vi "NML Data Acquisition-New.vi"() -> ()   [LabVIEW 2019]
doc: "This VI is designed to scan data each time the the trigger channel changes by an amount ∆ trigger.\nCopyright 2013\nScott Hannahs, NHMFL - FSU, July 2013"
uses:
  Sub Controls/Data Graph.ctl
  Sub Controls/Pause Switch.ctl
  Sub Controls/SystemCheckBox-resize.ctl
  Sub Controls/DataAcq User Events.ctl
panel:
  in  "Show Times":bool
  out "Time (mS)":dbl[](array[numeric])
  out "Logo":u16(ring)=2
  in  "ColorSelector":bool[](array[boolean])
  out "File Ref Num":refnum<file>
  out "All Data":dbl[][](array[numeric])
  out "Data":dbl[](array[numeric])=[nan, nan] format="%_4e"
  in  "Labels":string[](array[string])=["Field", "Timestamp"]
  out "Colors":u32[](array[colorbox])=[16748168, 2796287]
  out "# Data Points":i32
  in  "Comments":string="This data's for you!\n"
  in  "User Name":string="Conan The Scientist"
  in  "File Name":string="Test"
  in  "Open BD":bool
  in  "Pause":T1=TRUE
  in  "∆ Trigger":dbl min=0.0 format="%.3f"
  in  "Trigger Column":u32(ring) items=["Time", "Field", "Timestamp"]
  in  "Print":bool
  in  "Quit":bool
  in  "New/Stop":bool
  in  "Test":bool
  in  "Show Help":bool
  in  "Configure":bool
  in  "X-Axis":u32(ring)=1 items=["Point #", "Field", "Timestamp"]
  out "Data Plot":T2
  in  "Offset":dbl[](array[numeric])=[0.0, 0.0] format="%^_3e"
  in  "Display":T3[](array[typedef])=[TRUE, TRUE]
  in  "Scale":dbl[](array[numeric])=[1.0, 1.0] format="%^_3e"
  out "Status":string="Standby"
  # "NHMFL Data Acqusition System V 2.4.1\nScott Hannahs"
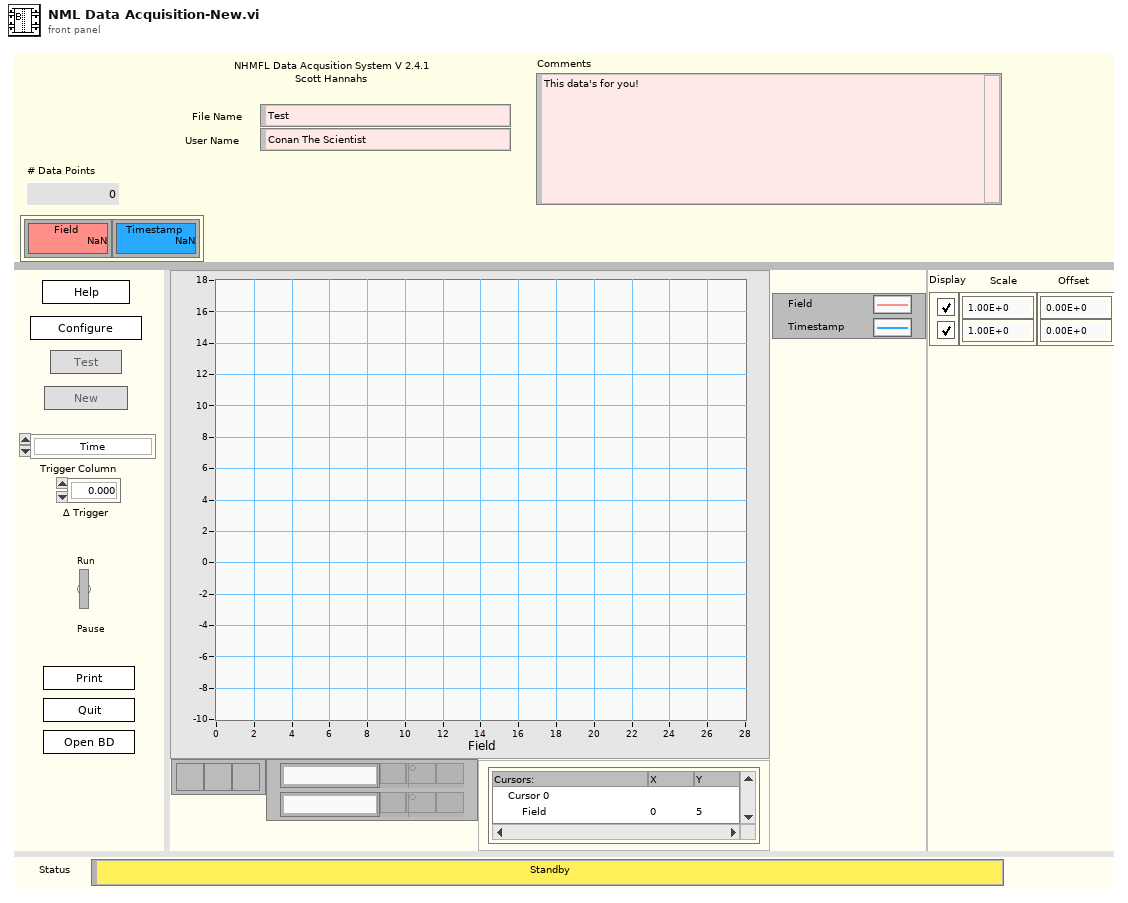
[diagram p1: front panel]
types:
  T1 = typedef "Pause Switch.ctl" = bool
  T2 = typedef "Data Graph.ctl" = cluster{dbl[], dbl[]}[]
  T3 = typedef "SystemCheckBox-resize.ctl" = bool
  T4 = typedef "DataAcq User Events.ctl" = enum16{"Update Data Display", "Store Data"}
  T5 = enum8{"Enabled", "Disabled", "Disabled and Grayed Out"}
  T6 = typedef "Instrument Properties.ctl" = cluster{"Public":T7, "Private":T8}
  T7 = typedef "Public.ctl" = cluster{"Column Name":string[], "Trace Color":u32[]}
  T8 = typedef "Private.ctl" = cluster{"Path":path, "VI Refnum":T9, "Name":string, "# of Values":i32, "Scale Factors":dbl[], "Display":T3[], "Offset":dbl[]}
  T9 = typedef "Instrument Ref.ctl" = refnum<vi>
  T10 = typedef "LVRectTypeDef.ctl" = cluster{"Left":i16, "Top":i16, "Right":i16, "Bottom":i16}
  T11 = typedef "LVPositionTypeDef.ctl" = cluster{"Left":i32, "Top":i32}
  T12 = typedef "imagedata.ctl" = cluster{"image type":i32, "image depth":i32, "image":u8[], "mask":u8[], "colors":u32[], "Rectangle":cluster{"left":i16, "top":i16, "right":i16, "bottom":i16}}
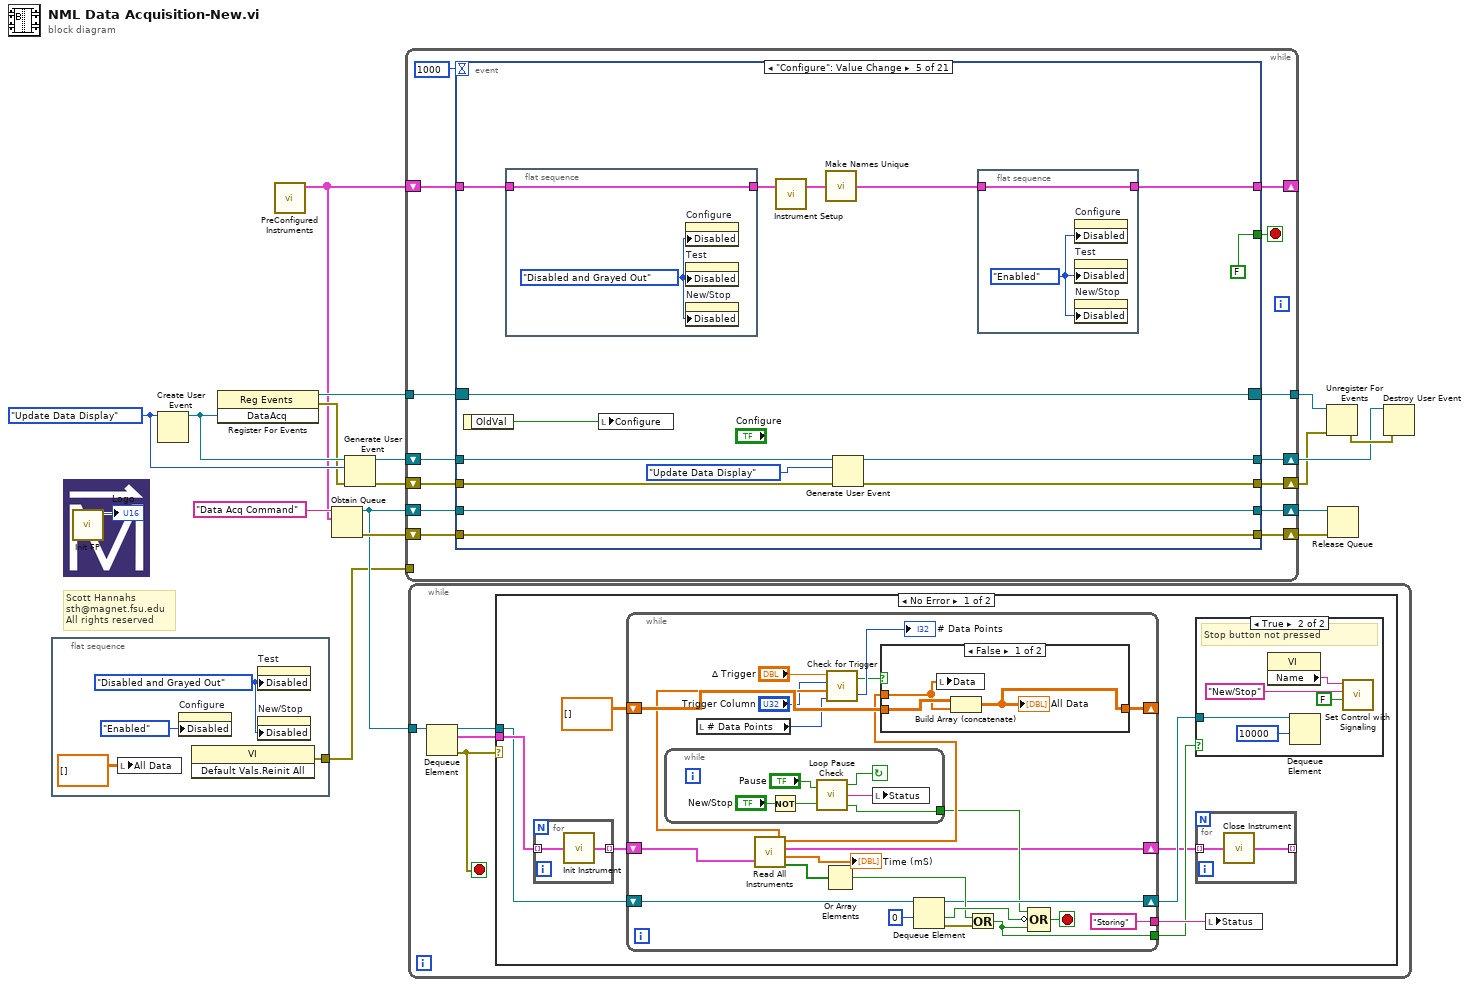
[diagram p0: block diagram]
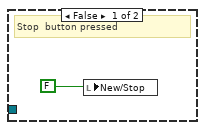
[diagram p2: hidden frame]
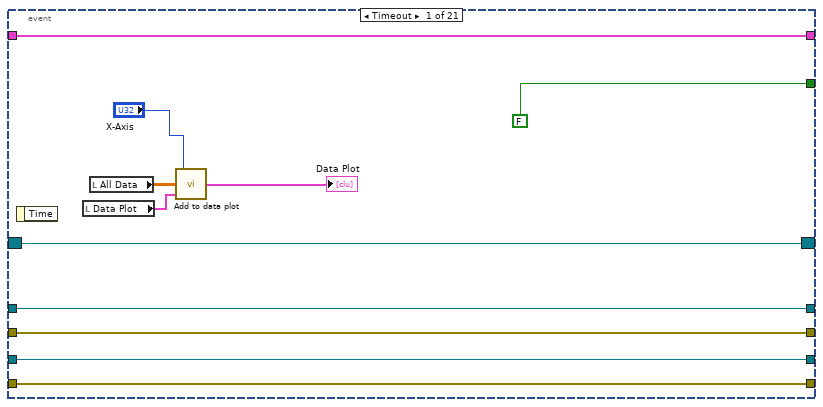
[diagram p5: hidden frame]
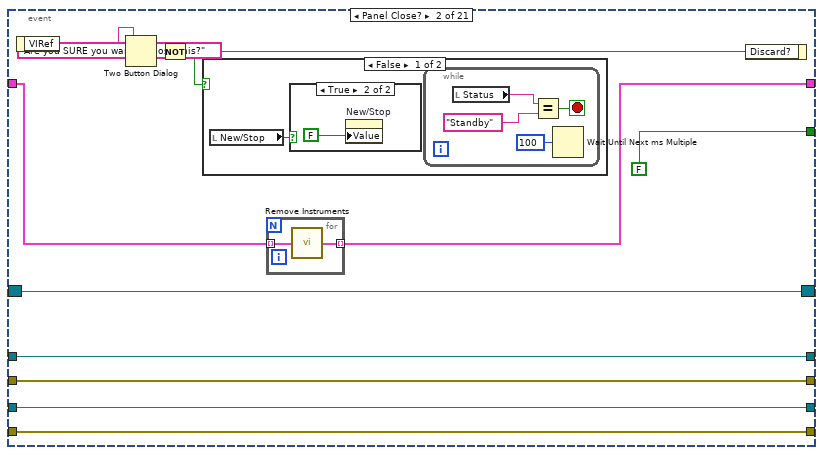
[diagram p6: hidden frame]
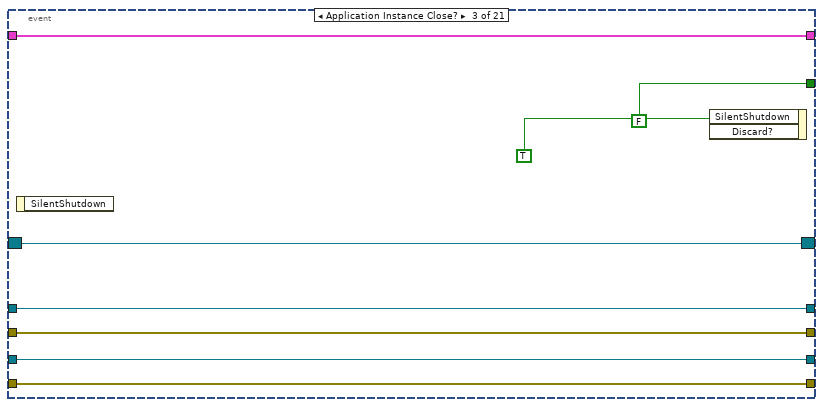
[diagram p9: hidden frame]
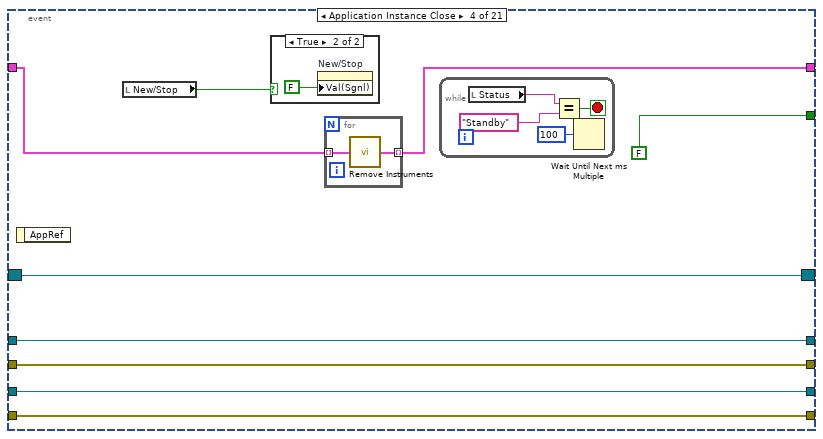
[diagram p10: hidden frame]
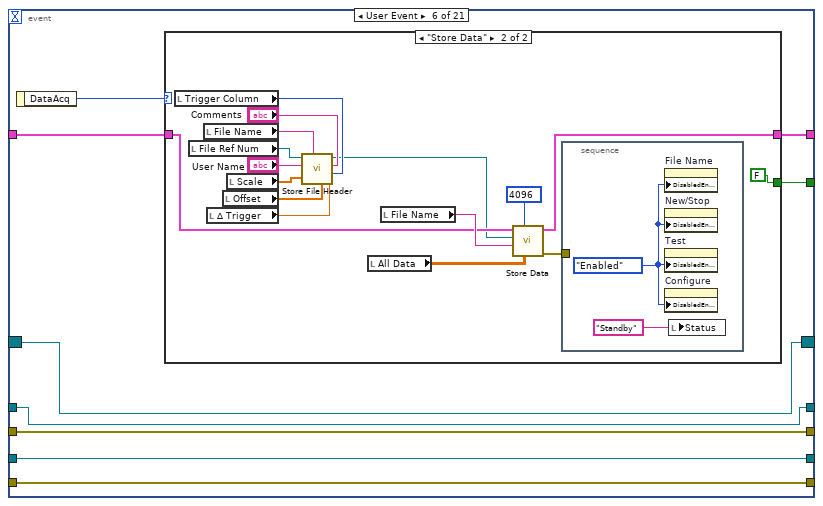
[diagram p12: hidden frame]
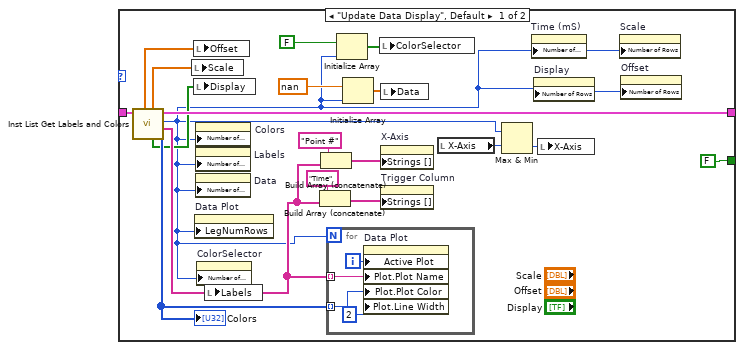
[diagram p13: hidden frame]
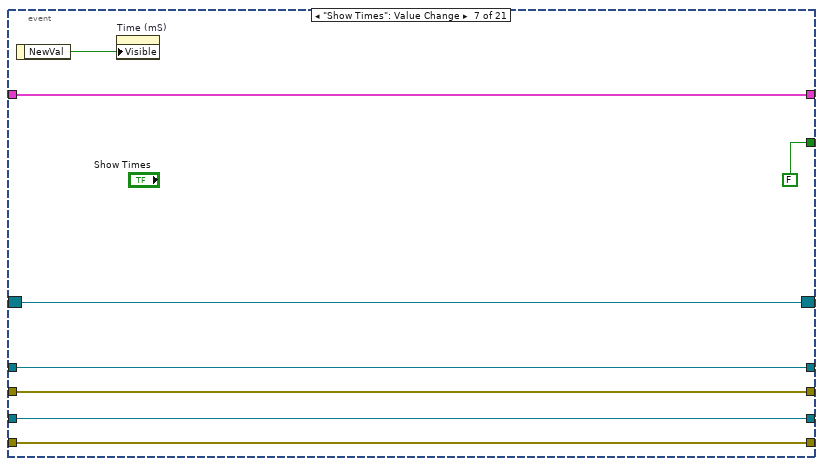
[diagram p14: hidden frame]
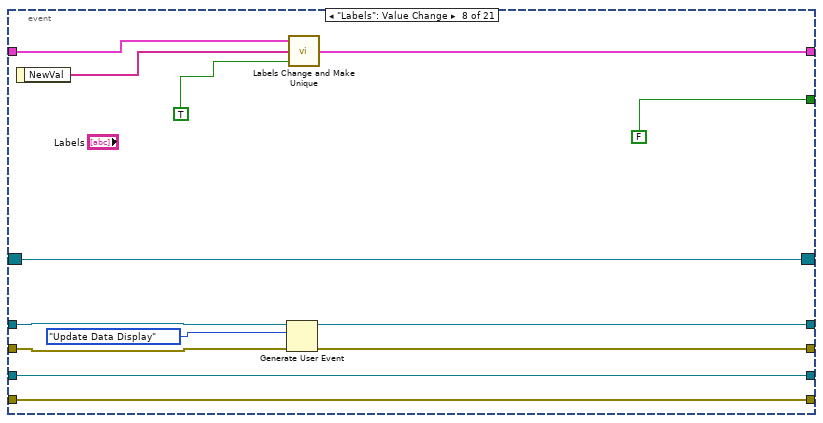
[diagram p15: hidden frame]
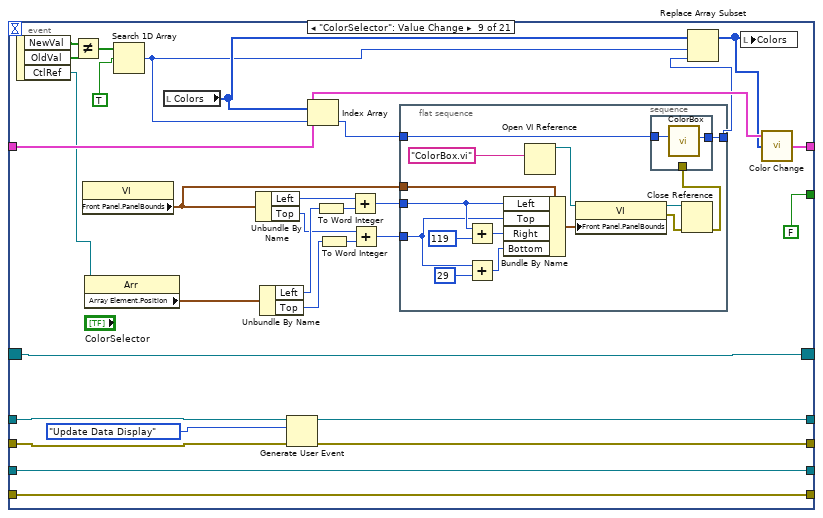
[diagram p16: hidden frame]
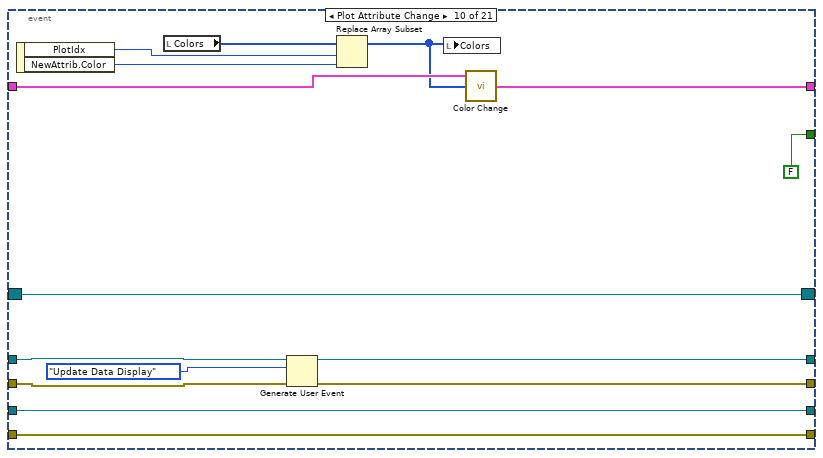
[diagram p17: hidden frame]
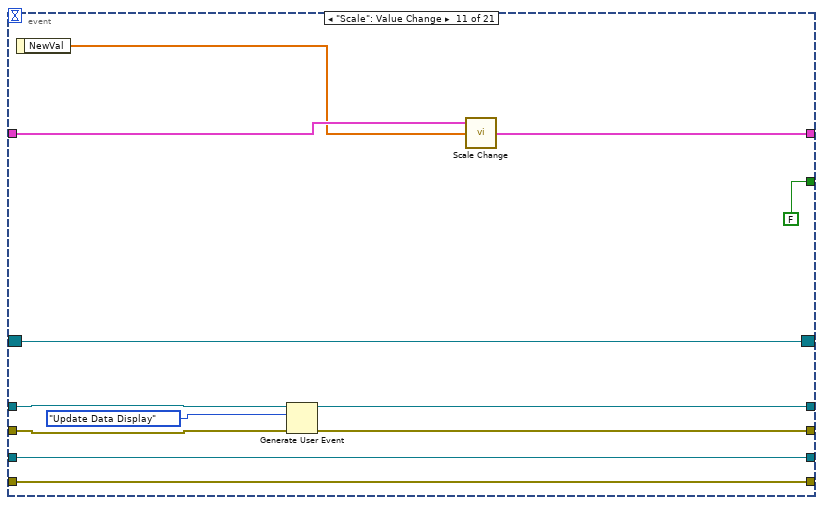
[diagram p18: hidden frame]
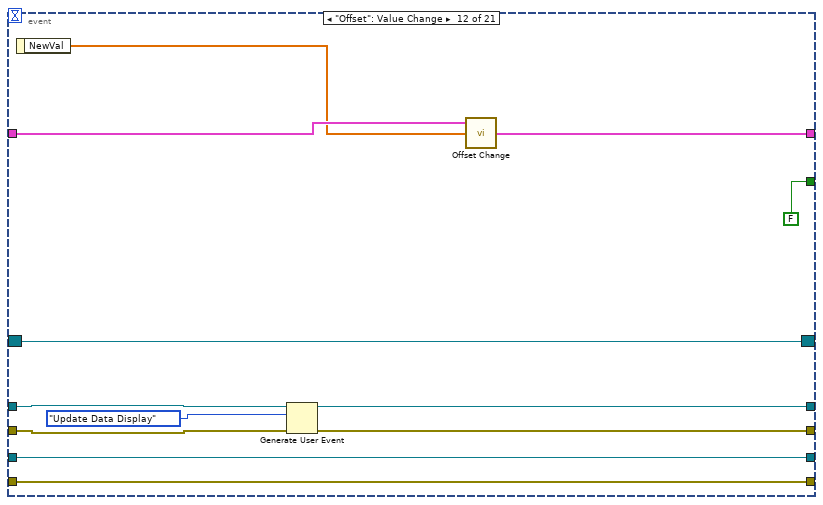
[diagram p19: hidden frame]
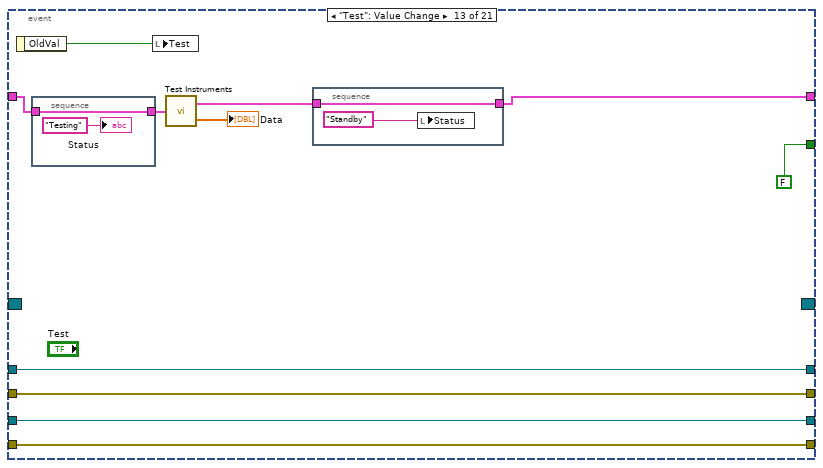
[diagram p20: hidden frame]
diagram:
  w16 = DataAcq_User_Events."Update Data Display" ("DataAcq")
  # "Scott Hannahs\nsth@magnet.fsu.edu\nAll rights reserved"
  n1 = flat-sequence {
    tunnel: [w21] -> w3
    frame #0 {
      w22 = T5."Disabled and Grayed Out" ("Disabled")
      n2 = local write "All Data"(dbl[][] [] ("All Data")) -> ()
      n3 = property on="Configure" class="Bool (strict)"("Disabled"=T5."Enabled") -> ()  [unwired: 2 in, 2 out]
      n4 = invoke class="VI" method="Default Vals.Reinit All"() -> (error out=w21:errorcluster)  [unwired: 3 in, 2 out]
      n5 = property on="Test" class="Bool (strict)"("Disabled"=w22) -> ()  [unwired: 2 in, 2 out]
      n6 = property on="New/Stop" class="Bool (strict)"("Disabled"=w22) -> ()  [unwired: 2 in, 2 out]
    }
  }
  n7 = call "Init FP.vi"() -> ("Logo"=→"Logo":u16)  [unwired: 11 in]
  n8 = Create User Event(user event datatype=w16) -> (user event=w17:refnum<user-event>)  [unwired: 1 in, 1 out]
  n9 = register-events(w17) -> (reference out=w18:refnum<event-registration>, error out=w15:errorcluster)  [unwired: 2 in]
  n10 = call "PreConfigured Instruments.vi"() -> ("PreConfigured Instruments"=w1:T6[])  [unwired: 11 in]
  n11 = Obtain Queue(name (unnamed)="Data Acq Command", element data type=w1) -> (queue out=w5:refnum<queue>, error out=w7:errorcluster)  [unwired: 3 in, 1 out]
  n12 = Generate User Event(user event=w17, event data cluster=w16, error in=w15) -> (user event out=w14:refnum<user-event>, error out=w9:errorcluster)  [unwired: 1 in]
  n13 = while {
    shift-right: [w35] -> _
    shift-left: w1 -> [w34]
    tunnel: w18 -> [w33]
    shift-right: [w31] -> w11
    shift-left: w14 -> [w32]
    tunnel: [w30] -> w13
    shift-right: [w28] -> w10
    shift-left: w5 -> [w29]
    shift-right: [w26] -> w8
    shift-left: w9 -> [w27]
    shift-right: [w24] -> w6
    shift-left: w7 -> [w25]
    tunnel: w3 -> [_]
    stop <- w36 stop-if-true
    n14 = event shown="[4] \"Configure\": Value Change" {
      selector: w33 -> [w38 w48 w67 w75 w96 w110 w164 w176 w209 w241 w253 w265 _ w288 w356 w365 w383 w398 w435 w444 w461]
      dyn-events: [w38 w48 w67 w75 w96 w110 w164 w176 w209 w241 w253 w265 _ w288 w356 w365 w383 w398 w435 w444 w461] -> w30
      timeout: 1000 -> [_ _ _ _ _ _ _ _ _ _ _ _ _ _ _ _ _ _ _ _ _]
      tunnel: [FALSE ("NewVal") FALSE ("NewVal") FALSE ("NewVal") FALSE ("NewVal") FALSE ("stop") w118 FALSE ("NewVal") FALSE ("NewVal") FALSE ("NewVal") FALSE ("NewVal") FALSE ("NewVal") FALSE ("NewVal") FALSE ("stop") FALSE ("stop") FALSE ("stop") FALSE ("stop") FALSE ("stop") FALSE ("NewVal") FALSE ("NewVal") w443 FALSE ("NewVal")] -> w36
      tunnel: w34 -> [w41 w54 w68 w77 w95 w116 w166 w180 w197 w233 w245 w257 w273 w292 w357 w371 w382 w408 w440 w450 w463]
      tunnel: [w41 w53 w68 w76 w92 w117 w166 w178 w211 w243 w255 w267 w270 w291 w357 w371 w381 w408 w440 w449 w463] -> w35
      tunnel: w32 -> [w45 w52 w72 w81 w104 w115 w163 w171 w205 w237 w249 w261 w277 w296 w359 w373 w390 w404 w439 w448 w460]
      tunnel: [w45 w52 w72 w81 w102 w115 w163 w170 w204 w236 w248 w260 w277 w295 w359 w373 w390 w404 w439 w448 w460] -> w31
      tunnel: [w43 w50 w70 w79 w99 w113 w161 w175 w208 w240 w252 w264 w276 w293 w362 w375 w388 w406 w437 w446 w458] -> w28
      tunnel: w29 -> [w43 w50 w70 w79 w99 w113 w161 w175 w208 w240 w252 w264 w276 w294 w362 w375 w388 w406 w437 w446 w458]
      tunnel: [w44 w51 w71 w80 w101 w114 w162 w169 w203 w235 w247 w259 w275 w286 w360 w376 w389 w405 w438 w447 w459] -> w26
      tunnel: w27 -> [w44 w51 w71 w80 w100 w114 w162 w168 w202 w234 w246 w258 w275 w287 w360 w376 w389 w405 w438 w447 w459]
      tunnel: [w42 w49 w69 w78 w98 w112 w160 w174 w207 w239 w251 w263 w274 w289 w361 w374 w387 w407 w436 w445 w457] -> w24
      tunnel: w25 -> [w42 w49 w69 w78 w98 w112 w160 w174 w207 w239 w251 w263 w274 w290 w361 w374 w387 w407 w436 w445 w457]
      event Timeout {
        n15 = event-data() -> ()  [unwired: 1 in, 1 out]
        n16 = local read "Data Plot"() -> (w37:T2)
        n17 = local read "All Data"() -> (w47:dbl[][])
        n18 = call "Add to data plot.vi"("Data Plot In"=w37, "All Data"=w47, "X-Axis"="X-Axis") -> ("Data PlotOut"=→"Data Plot":T2)
      }
      event Panel Close? {
        n19 = event-data() -> ()  [unwired: 1 in, 1 out]
        n20 = Two Button Dialog(message="Are you SURE you want to close this?") -> (T button?=w58:bool)  [unwired: 2 in]
        n21 = Not(x=w58) -> (.not. x?=w56:bool)
        n22 = case shown="False" w56 {
          frame False {
            n23 = local read "New/Stop"() -> (w61:bool)
            n24 = case shown="True" w61 {
              frame False {
              }
              frame True {
                n25 = property on="New/Stop" class="Bool (strict)"("Value"=FALSE ("New/Stop")) -> ()  [unwired: 2 in, 2 out]
              }
            }
            n26 = while {
              stop <- w65 stop-if-true
              n27 = local read "Status"() -> (w66:string)
              n28 = Equal?(x=w66, y="Standby") -> (x = y?=w65:bool)
              n29 = Wait Until Next ms Multiple(millisecond multiple=u32 100) -> ()  [unwired: 1 out]
            }
          }
          frame True {
          }
        }
        n30 = for {
          tunnel: w54 -> [w60] mode=indexing
          tunnel: [w59] -> w53 mode=indexing
          n31 = call "Remove Instruments.vi"("Instrument Prop"=w60) -> ("Instrument Prop Out"=w59:T6)
        }
        n32 = event-data("Discard?"=w56) -> ()  [unwired: 1 in, 1 out]
      }
      event Application Instance Close? {
        n33 = event-data() -> ()  [unwired: 1 in, 1 out]
        n34 = event-data("SilentShutdown"=TRUE) -> ()  [unwired: 2 in, 1 out]
      }
      event Application Instance Close {
        n35 = event-data() -> ()  [unwired: 1 in, 1 out]
        n36 = local read "New/Stop"() -> (w83:bool)
        n37 = case shown="True" w83 {
          frame False {
          }
          frame True {
            n38 = property on="New/Stop" class="Bool (strict)"("Val(Sgnl)"=FALSE ("New/Stop")) -> ()  [unwired: 2 in, 2 out]
          }
        }
        n39 = for {
          tunnel: w77 -> [w85] mode=indexing
          tunnel: [w84] -> w76 mode=indexing
          n40 = call "Remove Instruments.vi"("Instrument Prop"=w85) -> ("Instrument Prop Out"=w84:T6)
        }
        n41 = while {
          stop <- w89 stop-if-true
          n42 = local read "Status"() -> (w90:string)
          n43 = Equal?(x=w90, y="Standby") -> (x = y?=w89:bool)
          n44 = Wait Until Next ms Multiple(millisecond multiple=u32 100) -> ()  [unwired: 1 out]
        }
      }
      event "Configure": Value Change {
        n45 = event-data() -> ("OldVal"=w91:bool)  [unwired: 1 in]
        n46 = flat-sequence {
          tunnel: [w107] -> w94
          tunnel: w95 -> [w107]
          frame #0 {
            w106 = T5."Disabled and Grayed Out" ("Disabled")
            n47 = property on="Configure" class="Bool (strict)"("Disabled"=w106) -> ()  [unwired: 2 in, 2 out]
            n48 = property on="Test" class="Bool (strict)"("Disabled"=w106) -> ()  [unwired: 2 in, 2 out]
            n49 = property on="New/Stop" class="Bool (strict)"("Disabled"=w106) -> ()  [unwired: 2 in, 2 out]
          }
        }
        n50 = local write "Configure"(w91) -> ()
        n51 = call "Instrument Setup.vi"("Configured Inst"=w94) -> ("Configured Inst dup"=w97:T6[])  [unwired: 2 in]
        n52 = call "Make Names Unique.vi"("Configured Inst"=w97) -> ("Configured Inst dup"=w93:T6[])
        n53 = Generate User Event(user event=w104, event data cluster=DataAcq_User_Events."Update Data Display" ("event data"), error in=w100) -> (user event out=w102:refnum<user-event>, error out=w101:errorcluster)  [unwired: 1 in]
        n54 = flat-sequence {
          tunnel: w93 -> [w109]
          tunnel: [w109] -> w92
          frame #0 {
            w108 = T5."Enabled" ("Disabled")
            n55 = property on="Configure" class="Bool (strict)"("Disabled"=w108) -> ()  [unwired: 2 in, 2 out]
            n56 = property on="Test" class="Bool (strict)"("Disabled"=w108) -> ()  [unwired: 2 in, 2 out]
            n57 = property on="New/Stop" class="Bool (strict)"("Disabled"=w108) -> ()  [unwired: 2 in, 2 out]
          }
        }
      }
      event User Event {
        n58 = event-data() -> ("DataAcq"=w111:T4)  [unwired: 1 in]
        n59 = case shown="\"Store Data\"" w111 {
          tunnel: [FALSE ("stop") FALSE ("stop")] -> w118
          tunnel: [w136 w146] -> w117
          tunnel: w116 -> [w135 w145]
          frame "Update Data Display", Default {
            n60 = call "Inst List Get Labels and Colors.vi"("Instrument List"=w135) -> ("Colors"=w132:u32[], "Labels"=w125:string[], "Number of Columns"=w119:u32, "Instrument List Out"=w136:T6[], "Display"=w121:T3[], "Scale Factors"=w122:dbl[], "Offsets"=w120:dbl[])  [unwired: 4 in]
            "Colors" <- w132
            n61 = local write "Scale"(w122) -> ()
            n62 = local write "Offset"(w120) -> ()
            n63 = local write "Display"(w121) -> ()
            n64 = property on="Data Plot" class="XYGraph (strict)"("LegNumRows"=w119) -> ()  [unwired: 2 in, 2 out]
            n65 = property on="Colors" class="Arr (strict)"("Number of Columns"=w119) -> ()  [unwired: 2 in, 2 out]
            n66 = property on="Labels" class="Arr (strict)"("Number of Columns"=w119) -> ()  [unwired: 2 in, 2 out]
            n67 = property on="Data" class="Arr (strict)"("Number of Columns"=w119) -> ()  [unwired: 2 in, 2 out]
            n68 = property on="ColorSelector" class="Arr"("Number of Columns"=w119) -> ()  [unwired: 2 in, 2 out]
            n69 = local write "Labels"(w125) -> ()
            n70 = Build Array (concatenate)("Time", w125) -> (w131:string[])
            n71 = Build Array (concatenate)("Point #", w125) -> (w129:string[])
            n72 = for {
              N: w119 -> [_]
              tunnel: w125 -> [w139] mode=indexing
              tunnel: w132 -> [w141] mode=indexing
              i -> [w140]
              n73 = property on="Data Plot" class="XYGraph (strict)"("Active Plot"=w140, "Plot.Plot Name"=w139, "Plot.Plot Color"=w141, "Plot.Line Width"=u8 2) -> ()  [unwired: 2 in, 2 out]
            }
            n74 = Initialize Array(FALSE, w119) -> (w123:bool[])
            n75 = Initialize Array(nan, w119) -> (w134:dbl[])
            n76 = local write "ColorSelector"(w123) -> ()
            n77 = local write "Data"(w134) -> ()
            n78 = property on="X-Axis" class="Ring (strict)"("Strings []"=w129) -> ()  [unwired: 2 in, 2 out]
            n79 = property on="Trigger Column" class="Ring (strict)"("Strings []"=w131) -> ()  [unwired: 2 in, 2 out]
            n80 = local read "X-Axis"() -> (w126:u32)
            n81 = Max & Min(x=w119, y=w126) -> (min(x,y)=w127:u32)  [unwired: 1 out]
            n82 = property on="Time (mS)" class="Arr (strict)"("Number of Columns"=w119) -> ()  [unwired: 2 in, 2 out]
            n83 = property on="Display" class="Arr (strict)"("Number of Rows"=w119) -> ()  [unwired: 2 in, 2 out]
            n84 = local write "X-Axis"(w127) -> ()
            n85 = property on="Scale" class="Arr (strict)"("Number of Rows"=w119) -> ()  [unwired: 2 in, 2 out]
            n86 = property on="Offset" class="Arr (strict)"("Number of Rows"=w119) -> ()  [unwired: 2 in, 2 out]
          }
          frame "Store Data" {
            n87 = local read "Trigger Column"() -> (w155:u32)
            n88 = local read "File Ref Num"() -> (w150:refnum<file>)
            n89 = local read "File Name"() -> (w151:string)
            n90 = local read "∆ Trigger"() -> (w147:dbl)
            n91 = local read "Offset"() -> (w142:dbl[])
            n92 = local read "Scale"() -> (w148:dbl[])
            n93 = call "Store File Header.vi"("∆ Trigger"=w147, "Trigger Column"=w155, "Comments"="Comments", "Offsets"=w142, "Scale Factors"=w148, "Output File Name"=w151, "User Name"="User Name", "File Ref Num In"=w150) -> ("File Ref Num"=w144:refnum<file>)  [unwired: 3 in]
            n94 = local read "All Data"() -> (w156:dbl[][])
            n95 = local read "File Name"() -> (w154:string)
            n96 = call "Store Data.vi"("All Data"=w156, "Block Size"=4096, "File Name"=w154, "Byte Stream File in"=w144, "Instrument List In"=w145) -> ("error out"=w149:errorcluster, "Instrument List Out"=w146:T6[])  [unwired: 5 in]
            n97 = stacked-sequence {
              tunnel: w149 -> [_]
              frame #0 {
                w158 = T5."Enabled" ("Disabled")
                n98 = property on="File Name" class="Str"("DisabledEnum"=w158) -> ()  [unwired: 2 in, 2 out]
                n99 = property on="New/Stop" class="Bool (strict)"("DisabledEnum"=w158) -> ()  [unwired: 2 in, 2 out]
                n100 = property on="Test" class="Bool (strict)"("DisabledEnum"=w158) -> ()  [unwired: 2 in, 2 out]
                n101 = property on="Configure" class="Bool (strict)"("DisabledEnum"=w158) -> ()  [unwired: 2 in, 2 out]
                n102 = local write "Status"("Standby") -> ()
              }
            }
          }
        }
      }
      event "Show Times": Value Change {
        n103 = event-data() -> ("NewVal"=w167:bool)  [unwired: 1 in]
        n104 = property on="Time (mS)" class="Arr (strict)"("Visible"=w167) -> ()  [unwired: 2 in, 2 out]
      }
      event "Labels": Value Change {
        n105 = event-data() -> ("NewVal"=w179:string[])  [unwired: 1 in]
        n106 = Generate User Event(user event=w171, event data cluster=DataAcq_User_Events."Update Data Display" ("event data"), error in=w168) -> (user event out=w170:refnum<user-event>, error out=w169:errorcluster)  [unwired: 1 in]
        n107 = call "Labels Change and Make Unique.vi"("Force Update"=TRUE, "Labels"=w179, "Configured Inst Input"=w180) -> ("Configured Inst dup"=w178:T6[])
      }
      event "ColorSelector": Value Change {
        n108 = event-data() -> ("NewVal"=w199:bool[], "OldVal"=w198:bool[], "CtlRef"=w186:refnum<vi>)  [unwired: 1 in]
        n109 = Not Equal?(x=w199, y=w198) -> (x != y?=w201:bool[])
        n110 = property class="VI"() -> ("Front Panel.PanelBounds"=w191:T10)  [unwired: 2 in, 2 out]
        n111 = property class="Arr"(reference=w186) -> ("Array Element.Position"=w196:T11)  [unwired: 1 in, 2 out]
        n112 = Search 1D Array(1D array=w201, element=TRUE) -> (index of element=w181:i32)  [unwired: 1 in]
        n113 = local read "Colors"() -> (w184:u32[])
        n114 = Unbundle By Name(w191) -> ("Left"=w195:i16, "Top"=w193:i16)
        n115 = Unbundle By Name(w196) -> ("Left"=w194:i32, "Top"=w192:i32)
        n116 = Generate User Event(user event=w205, event data cluster=DataAcq_User_Events."Update Data Display" ("event data"), error in=w202) -> (user event out=w204:refnum<user-event>, error out=w203:errorcluster)  [unwired: 1 in]
        n117 = Index Array(array=w184, index=w181) -> (element=w185:u32)
        n118 = To Word Integer(number=w194) -> (16bit integer=w190:i16)
        n119 = To Word Integer(number=w192) -> (16bit integer=w189:i16)
        n120 = Add(x=w195, y=w190) -> (x+y=w187:i16)
        n121 = Add(x=w193, y=w189) -> (x+y=w188:i16)
        n122 = flat-sequence {
          tunnel: w185 -> [w226]
          tunnel: [w225] -> w183
          tunnel: w191 -> [w221]
          tunnel: w187 -> [w220]
          tunnel: w188 -> [w217]
          frame #0 {
            n123 = Add(x=w220, y=i16 119) -> (x+y=w218:i16)
            n124 = Add(x=w217, y=i16 29) -> (x+y=w215:i16)
            n125 = Bundle By Name(cluster=w221, "Left"=w220, "Top"=w217, "Right"=w218, "Bottom"=w215) -> (w222:T10)
            n126 = Open VI Reference(vi path="ColorBox.vi") -> (vi reference=w224:refnum<vi>)  [unwired: 5 in, 1 out]
            n127 = property class="VI"(reference=w224, "Front Panel.PanelBounds"=w222) -> (reference out=w213:refnum<vi>, error out=w214:errorcluster)  [unwired: 1 in]
            n128 = Close Reference(reference=w213, error in (no error)=w214) -> (error out=w212:errorcluster)
            n129 = stacked-sequence {
              tunnel: w226 -> [w228]
              tunnel: [w227] -> w225
              tunnel: w212 -> [_]
              frame #0 {
                n130 = call "ColorBox.vi"("Color Box In"=w228) -> ("Color Box Out"=w227:u32)  [unwired: 10 in]
              }
            }
          }
        }
        n131 = Replace Array Subset(array=w184, new element=w183, index=w181) -> (w182:u32[])
        n132 = local write "Colors"(w182) -> ()
        n133 = call "Color Change.vi"("Colors"=w182, "Configured Inst Input"=w197) -> ("Configured Inst dup"=w211:T6[])  [unwired: 1 in]
      }
      event Plot Attribute Change {
        n134 = event-data() -> ("PlotIdx"=w230:i32, "NewAttrib.Color"=w229:u32)  [unwired: 1 in]
        n135 = local read "Colors"() -> (w232:u32[])
        n136 = Generate User Event(user event=w237, event data cluster=DataAcq_User_Events."Update Data Display" ("event data"), error in=w234) -> (user event out=w236:refnum<user-event>, error out=w235:errorcluster)  [unwired: 1 in]
        n137 = Replace Array Subset(array=w232, new element=w229, index=w230) -> (w231:u32[])
        n138 = local write "Colors"(w231) -> ()
        n139 = call "Color Change.vi"("Colors"=w231, "Configured Inst Input"=w233) -> ("Configured Inst dup"=w243:T6[])  [unwired: 1 in]
      }
      event "Scale": Value Change {
        n140 = event-data() -> ("NewVal"=w244:dbl[])  [unwired: 1 in]
        n141 = Generate User Event(user event=w249, event data cluster=DataAcq_User_Events."Update Data Display" ("event data"), error in=w246) -> (user event out=w248:refnum<user-event>, error out=w247:errorcluster)  [unwired: 1 in]
        n142 = call "Scale Change.vi"("Scale Factors"=w244, "Configured Inst Input"=w245) -> ("Configured Inst dup"=w255:T6[])  [unwired: 1 in]
      }
      event "Offset": Value Change {
        n143 = event-data() -> ("NewVal"=w256:dbl[])  [unwired: 1 in]
        n144 = Generate User Event(user event=w261, event data cluster=DataAcq_User_Events."Update Data Display" ("event data"), error in=w258) -> (user event out=w260:refnum<user-event>, error out=w259:errorcluster)  [unwired: 1 in]
        n145 = call "Offset Change.vi"("Offsets"=w256, "Configured Inst Input"=w257) -> ("Configured Inst dup"=w267:T6[])  [unwired: 1 in]
      }
      event "Test": Value Change {
        n146 = event-data() -> ("OldVal"=w268:bool)  [unwired: 1 in]
        n147 = stacked-sequence {
          tunnel: w273 -> [w281]
          tunnel: [w281] -> w272
          frame #0 {
            "Status" <- "Testing"
          }
        }
        n148 = local write "Test"(w268) -> ()
        n149 = call "Test Instruments.vi"("Instrument List In"=w272) -> ("Instrument List Out"=w271:T6[], "Test Data"=→"Data":dbl[])
        n150 = stacked-sequence {
          tunnel: [w279] -> w270
          tunnel: w271 -> [w279]
          frame #0 {
            n151 = local write "Status"("Standby") -> ()
          }
        }
      }
      event "New/Stop": Value Change {
        n152 = event-data() -> ("OldVal"=w284:bool, "NewVal"=w285:bool)  [unwired: 1 in]
        n153 = Exclusive Or(1:w285, 2:w284) -> (0:w283:bool)
        n154 = case shown="True" w283 {
          tunnel: w296 -> [w299 w313]
          tunnel: [w299 w312] -> w295
          tunnel: w294 -> [w301 w311]
          tunnel: [w301 w310] -> w293
          tunnel: w292 -> [w302 w309]
          tunnel: [w302 w308] -> w291
          tunnel: w290 -> [w300 w307]
          tunnel: [w300 w306] -> w289
          tunnel: w287 -> [w298 w305]
          tunnel: [w298 w304] -> w286
          tunnel: w285 -> [_ w303]
          frame False {
          }
          frame True {
            n155 = case shown="True" w303 {
              tunnel: [w323 w332] -> w312
              tunnel: w313 -> [w320 w333]
              tunnel: w311 -> [w318 w340]
              tunnel: [w318 w339] -> w310
              tunnel: w309 -> [w319 w338]
              tunnel: [w319 w338] -> w308
              tunnel: [w321 w337] -> w306
              tunnel: w307 -> [w317 w336]
              tunnel: w305 -> [w314 w331]
              tunnel: [w314 w330] -> w304
              frame False {
                n156 = while {
                  tunnel: [w325] -> w316
                  tunnel: w317 -> [w325]
                  stop <- w324 stop-if-true
                  n157 = local read "Status"() -> (w328:string)
                  n158 = Equal?(x=w328, y="Storing") -> (x = y?=w324:bool)
                  n159 = Wait Until Next ms Multiple(millisecond multiple=u32 100) -> ()  [unwired: 1 out]
                }
                n160 = property on="New/Stop" class="Bool (strict)"("DisabledEnum"=T5."Disabled and Grayed Out" ("Disabled")) -> ()  [unwired: 2 in, 2 out]
                n161 = Generate User Event(user event=w320, event data cluster=DataAcq_User_Events."Store Data" ("event data"), error in=w316) -> (user event out=w323:refnum<user-event>, error out=w321:errorcluster)  [unwired: 1 in]
              }
              frame True {
                n162 = call "Get Shared Data Dir.vi"() -> ("Data Directory Path"=w344:path)  [unwired: 2 in, 1 out]
                n163 = call "Open Next Numbered File.vi"("Dir Path"=w344, "Input File Pattern"="File Name") -> ("Stop"=w341:bool, "Output File Name"=w335:string, "refnum out"=→"File Ref Num":refnum<file>)  [unwired: 3 in, 1 out]
                n164 = local write "File Name"(w335) -> ()
                n165 = local write "Data Plot"(T2 [] ("Data Plot")) -> ()
                n166 = local write "# Data Points"(0 ("# Data Points")) -> ()
                n167 = case shown="False" w341 {
                  tunnel: w340 -> [w352 w354]
                  tunnel: [w350 w354] -> w339
                  tunnel: w338 -> [w351 _]
                  tunnel: [w349 w353] -> w337
                  tunnel: w336 -> [w348 w353]
                  frame False {
                    w347 = T5."Disabled and Grayed Out" ("Disabled")
                    n168 = Enqueue Element(queue=w352, element=w351, error in (no error)=w348) -> (queue out=w350:refnum<queue>, error out=w349:errorcluster)  [unwired: 1 in, 1 out]
                    n169 = property on="File Name" class="Str"("DisabledEnum"=w347) -> ()  [unwired: 2 in, 2 out]
                    n170 = property on="Test" class="Bool (strict)"("DisabledEnum"=w347) -> ()  [unwired: 2 in, 2 out]
                    n171 = property on="Configure" class="Bool (strict)"("DisabledEnum"=w347) -> ()  [unwired: 2 in, 2 out]
                  }
                  frame True {
                    n172 = local write "New/Stop"(FALSE ("New/Stop")) -> ()
                  }
                }
                n173 = Generate User Event(user event=w333, event data cluster=DataAcq_User_Events."Update Data Display" ("event data"), error in=w331) -> (user event out=w332:refnum<user-event>, error out=w330:errorcluster)  [unwired: 1 in]
                n174 = local write "All Data"(dbl[][] [] ("All Data")) -> ()
              }
            }
          }
        }
      }
      event "Show Help": Value Change {
        n175 = event-data() -> ("NewVal"=w363:bool)  [unwired: 1 in]
        n176 = Control Help Window(1:w363) -> ()  [unwired: 1 in]
      }
      event "Print": Value Change {
        n177 = event-data() -> ("OldVal"=w364:bool)  [unwired: 1 in]
        n178 = local write "Print"(w364) -> ()
        n179 = local read "X-Axis"() -> (w368:u32)
        n180 = property on="X-Axis" class="Ring (strict)"() -> ("Strings []"=w369:string[])  [unwired: 2 in, 2 out]
        n181 = invoke on="Data Plot" class="XYGraph (strict)" method="Get Image"("image depth"=32 ("Image Depth"), "bg color"=u32 16448250) -> ("image data"=w367:T12)  [unwired: 4 in, 5 out]
        n182 = local read "Comments"() -> (w377:string)
        n183 = local read "File Name"() -> (w378:string)
        n184 = Index Array(array=w369, index=w368) -> (element=w366:string)
        n185 = call "Print Data Plot.vi"("X-Axis"=w366, "image data"=w367, "File Name"=w378, "Comments"=w377) -> ()  [unwired: 5 in]
      }
      event "Display": Value Change {
        n186 = event-data() -> ("NewVal"=w380:T3[])  [unwired: 1 in]
        n187 = local read "X-Axis"() -> (w385:u32)
        n188 = Decrement(x=w385) -> (x-1=w384:u32)
        n189 = for {
          tunnel: w380 -> [w394] mode=indexing
          tunnel: w384 -> [w397]
          i -> [w396]
          n190 = To Unsigned Long Integer(number=w396) -> (unsigned 32bit integer=w391:u32)
          n191 = Not Equal?(x=w391, y=w397) -> (x != y?=w395:bool)
          n192 = Select(t=w394, s=w395, f=T3 FALSE) -> (s? t:f=w393:T3)
          n193 = property on="Data Plot" class="XYGraph (strict)"("Active Plot"=w391, "Plot.Visible?"=w393) -> ()  [unwired: 2 in, 2 out]
        }
        n194 = call "Display Change.vi"("Display"=w380, "Configured Inst Input"=w382) -> ("Configured Inst dup"=w381:T6[])  [unwired: 3 in]
      }
      event "X-Axis": Value Change {
        n195 = event-data() -> ("NewVal"=w414:u32, "OldVal"=w403:u32)  [unwired: 1 in]
        n196 = local read "Data Plot"() -> (w412:T2)
        n197 = Decrement(x=w403) -> (x-1=w401:u32)
        n198 = Decrement(x=w414) -> (x-1=w399:u32)
        n199 = Greater Or Equal To 0?(x=w401) -> (x >= 0?=w402:bool)
        n200 = Greater Or Equal To 0?(x=w399) -> (x >= 0?=w400:bool)
        n201 = call "Generate X Axis.vi"("Axis Index"=w399, "Data Plot"=w412) -> ("X Axis"=w411:dbl[])
        n202 = Array Size(array=w412) -> (size(s)=w413:i32)
        n203 = case shown="True" w402 {
          tunnel: w401 -> [_ w418]
          frame False {
          }
          frame True {
            n204 = local read "Display"() -> (w420:T3[])
            n205 = Index Array(array=w420, index=w418) -> (element=w419:T3)
            n206 = To Unsigned Long Integer(number=w418) -> (unsigned 32bit integer=w417:u32)
            n207 = property on="Data Plot" class="XYGraph (strict)"("Active Plot"=w417, "Plot.Visible?"=w419) -> ()  [unwired: 2 in, 2 out]
          }
        }
        n208 = case shown="True" w400 {
          tunnel: w399 -> [_ w416]
          frame False {
          }
          frame True {
            n209 = property on="Data Plot" class="XYGraph (strict)"("Active Plot"=w416, "Plot.Visible?"=FALSE ("Plot.Visible")) -> ()  [unwired: 2 in, 2 out]
          }
        }
        n210 = for {
          N: w413 -> [_]
          shift-right: [w424] -> w410
          shift-left: w412 -> [w423]
          tunnel: w411 -> [w425]
          i -> [w421]
          n211 = Index Array(array=w423, index=w421) -> (element=w427:cluster{dbl[], dbl[]})
          n212 = Unbundle(w427) -> (w426:dbl[])  [unwired: 1 out]
          n213 = Bundle("X Axis"=w425, w426) -> (w422:cluster{"X Axis":dbl[], dbl[]})  [unwired: 1 in]
          n214 = Replace Array Subset(array=w423, new element=w422, index=w421) -> (w424:T2)
        }
        n215 = local write "Data Plot"(w410) -> ()
      }
      event Pane Size {
        w430 = 12 ("Named Numeric Size:Height")
        n216 = event-data() -> ()  [unwired: 1 in, 1 out]
        n217 = invoke on="Data Plot" class="XYGraph (strict)" method="FitControlToPane"() -> (error out=w433:errorcluster)  [unwired: 3 in, 2 out]
        n218 = property on="Data Plot" class="XYGraph (strict)"(error in=w433) -> ("Plot Bounds"=w434:T10)  [unwired: 1 in, 2 out]
        n219 = Unbundle By Name(w434) -> ("Bottom"=w432:i16)
        n220 = To Long Integer(number=w432) -> (32bit integer=w428:i32)
        n221 = To Unsigned Long Integer(number=w430) -> (unsigned 32bit integer=w429:u32)
        n222 = Add(x=w430, y=w428) -> (x+y=w431:i32)
        n223 = property on="X-Axis" class="Ring (strict)"("Height"=w429, "Top"=w431) -> ()  [unwired: 2 in, 2 out]
      }
      event "Quit": Value Change {
        n224 = event-data() -> ("NewVal"=w443:bool)  [unwired: 1 in]
        n225 = Not(x=w443) -> (.not. x?=w442:bool)
        n226 = local write "Quit"(w442) -> ()
        n227 = for {
          tunnel: w450 -> [w452] mode=indexing
          tunnel: [w451] -> w449 mode=indexing
          n228 = call "Remove Instruments.vi"("Instrument Prop"=w452) -> ("Instrument Prop Out"=w451:T6)
        }
      }
      event "Open BD": Value Change {
        n229 = event-data() -> ("OldVal"=w453:bool)  [unwired: 1 in]
        n230 = local write "Open BD"(w453) -> ()
        n231 = Current VI's Path() -> (path=w456:path)
        n232 = Open VI Reference(vi path=w456) -> (vi reference=w455:refnum<vi>)  [unwired: 5 in, 1 out]
        n233 = invoke class="VI" method="BD.OpenInNativeWind"(reference=w455, "Host Window"=u64 0) -> ()  [unwired: 4 in, 6 out]
      }
    }
  }
  n234 = while {
    tunnel: w5 -> [w467]
    stop <- w466 stop-if-true
    n235 = Dequeue Element(queue=w467) -> (queue out=w465:refnum<queue>, element=w464:T6[], error out=w466:errorcluster)  [unwired: 2 in, 1 out]
    n236 = case shown="No Error" w466 {
      tunnel: w465 -> [w472 _]
      tunnel: w464 -> [w475 _]
      frame No Error {
        n237 = for {
          tunnel: w475 -> [w517] mode=indexing
          tunnel: [w516] -> w474 mode=indexing
          n238 = call "Init Instrument.vi"("Instrument Prop"=w517) -> ("Instrument Prop 2"=w516:T6)
        }
        n239 = while {
          shift-right: [w503] -> _
          shift-left: dbl[][] [] ("Array 2") -> [w502]
          tunnel: ["Storing" ("y")] -> w471
          tunnel: [w487] -> w470
          shift-right: [w484] -> w468
          shift-left: w474 -> [w505]
          shift-right: [w488] -> w469
          shift-left: w472 -> [w501]
          stop <- w491 stop-if-true
          n240 = while {
            tunnel: [w510] -> w486
            stop <- w514 continue-if-true
            n241 = Not(x="New/Stop") -> (.not. x?=w513:bool)
            n242 = call "Loop Pause Check.vi"("Pause"="Pause", "Stop"=w513) -> ("Pause"=w514:bool, "State"=w512:string, "ABORT"=w510:bool)
            n243 = local write "Status"(w512) -> ()
          }
          n244 = local read "# Data Points"() -> (w495:i32)
          n245 = call "Read All Instruments.vi"("Instrument Array In"=w505) -> ("Data Array"=w499:dbl[], "Instrument Array Out"=w484:T6[], "Time (mS)"=→"Time (mS)":dbl[], "Instrument Stop"=w504:bool[])  [unwired: 1 in]
          n246 = Or Array Elements(Boolean array=w504) -> (logical OR=w490:bool)
          n247 = call "Check for Trigger.vi"("# Data Points"=w495, "Current Values"=w499, "Trigger Column"="Trigger Column", "Æ Trigger Value"="∆ Trigger") -> ("# Data Points Out"=→"# Data Points":i32, "Wait"=w494:bool)
          n248 = case shown="False" w494 {
            tunnel: [w508 w509] -> w503
            tunnel: w502 -> [w507 w509]
            tunnel: w499 -> [w506 _]
            frame False {
              n249 = local write "Data"(w506) -> ()
              n250 = Build Array (concatenate)(w507, w506) -> (w508:dbl[][])
              "All Data" <- w508
            }
            frame True {
            }
          }
          n251 = Dequeue Element(queue=w501, timeout in ms (-1)=0) -> (queue out=w488:refnum<queue>, timed out?=w492:bool, error out=w489:errorcluster)  [unwired: 1 in, 1 out]
          n252 = Or(x=w490, y=w489) -> (x .or. y?=w487:bool)
          n253 = Compound Arithmetic op=OR(w486, invert w492, w487) -> (w491:bool)
        }
        n254 = case shown="True" w470 {
          tunnel: w469 -> [_ w478]
          frame False {
            # "Stop  button pressed"
            n255 = local write "New/Stop"(FALSE ("New/Stop")) -> ()
          }
          frame True {
            # "Stop button not pressed"
            n256 = property class="VI"() -> ("Name"=w480:string)  [unwired: 2 in, 2 out]
            n257 = Dequeue Element(queue=w478, timeout in ms (-1)=10000) -> ()  [unwired: 1 in, 4 out]
            n258 = call "Set Control with Signaling.vi"("Value"=FALSE ("New/Stop"), "Control Name"="New/Stop", "VI Name"=w480) -> ()  [unwired: 8 in, 1 out]
          }
        }
        n259 = for {
          tunnel: w468 -> [w483] mode=indexing
          tunnel: [w482] -> _ mode=indexing
          n260 = call "Close Instrument.vi"("Instrument Prop"=w483) -> ("Instrument Prop 2"=w482:T6)
        }
        n261 = local write "Status"(w471) -> ()
      }
      frame Error {
      }
    }
  }
  n262 = Unregister For Events(event registration refnum=w13, error in=w8) -> (error out=w12:errorcluster)
  n263 = Release Queue(queue=w10, error in (no error)=w6) -> ()  [unwired: 1 in, 3 out]
  n264 = Destroy User Event(user event=w11, error in=w12) -> ()  [unwired: 1 out]
